vi "N5700 Error Query.vi"(0 "VISA":refnum<visa-resource-name>, 11 "error":errorcluster) -> (4 "VISA out":refnum<visa-resource-name>, 8 "Error Number":i32, 10 "Error Message":string, 15 "error out":errorcluster)   [LabVIEW 2020]
doc: "This VI reads an error code and a message from the instrument's error queue (query SYST:ERR?\"). The instrument error is cast to be within the range allowed for VISA custom errors. See \"Agilent N5700 Readme.html\" file for description of custom error codes\n\nNote: This VI is called automatically by most driver VIs so it is not usually necessary to call this in an application."
panel:
  # "Agilent Technologies  \nSeries N5700A\n  DC Power Supplies"
  # "Read\n  SYSTEM:ERROR?"
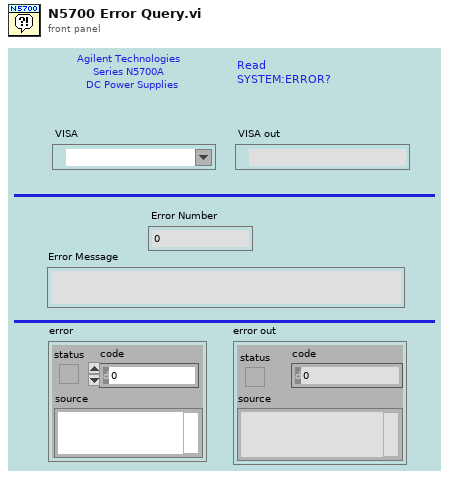
[diagram p1: front panel]
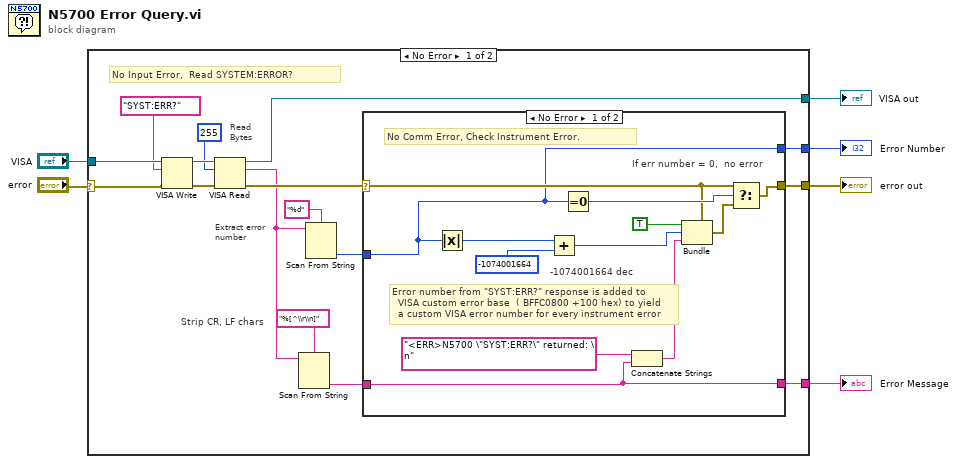
[diagram p0: block diagram]
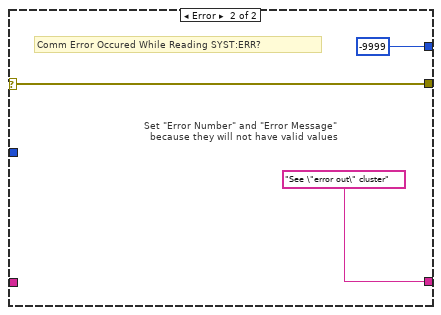
[diagram p2: hidden frame]
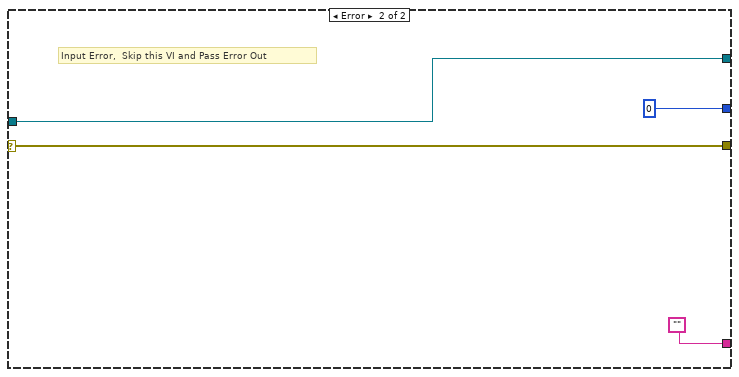
[diagram p3: hidden frame]
diagram:
  n1 = case shown="No Error" "error" {
    selector: "error" -> [w7 w38]
    tunnel: [w22 ""] -> w6
    tunnel: [w21 0] -> w5
    tunnel: [w20 w41] -> w4
    tunnel: "VISA" -> [w19 w41]
    tunnel: [w8 w38] -> w2
    frame No Error {
      # "No Input Error,  Read SYSTEM:ERROR?"
      # "Extract error\nnumber"
      # "Read\nBytes"
      # "Strip CR, LF chars"
      n2 = VISA Write(VISA resource name=w19, write buffer="SYST:ERR?", error in (no error)=w7) -> (VISA resource name out=w18:refnum<visa-resource-name>, error out=w16:errorcluster)  [unwired: 1 out]
      n3 = VISA Read(VISA resource name=w18, byte count=u32 255 ("byte count (0)"), error in (no error)=w16) -> (VISA resource name out=w20:refnum<visa-resource-name>, read buffer=w10:string, error out=w13:errorcluster)  [unwired: 1 out]
      n4 = Scan From String(format string="%[^\\r\\n]", input string=w10) -> (output 1=w9:string)  [unwired: 3 in, 3 out]
      n5 = Scan From String(format string="%d", input string=w10) -> (output 1=w14:i32)  [unwired: 3 in, 3 out]
      n6 = case shown="No Error" w13 {
        selector: w13 -> [w27 w36]
        tunnel: [w31 w36] -> w8
        tunnel: [w28 "See \"error out\" cluster" ("format string")] -> w22
        tunnel: [w26 -9999] -> w21
        tunnel: w14 -> [w26 _]
        tunnel: w9 -> [w28 _]
        frame No Error {
          # "No Comm Error, Check Instrument Error."
          # "Error number from \"SYST:ERR?\" response is added to \n  VISA custom error base  ( BFFC0800 +100 hex) to yield  \n  a custom VISA error number for every instrument error"
          # "-1074001664 dec"
          # "If err number = 0,  no error"
          n7 = Absolute Value(x=w26) -> (abs(x)=w25:i32)
          n8 = Add(x=w25, y=-1074001664) -> (x+y=w23:i32)
          n9 = Equal To 0?(x=w26) -> (x = 0?=w29:bool)
          n10 = Concatenate Strings("<ERR>N5700 \"SYST:ERR?\" returned: \n" ("Source"), w28) -> (w33:string)
          n11 = Bundle(cluster=w27, "status"=TRUE ("Status"), "code"=w23, "source"=w33) -> (w32:errorcluster)
          n12 = Select(t=w27, s=w29, f=w32) -> (s? t:f=w31:errorcluster)
        }
        frame Error {
          # "Set \"Error Number\" and \"Error Message\"\n  because they will not have valid values"
          # "Comm Error Occured While Reading SYST:ERR?"
        }
      }
    }
    frame Error {
      # "Input Error,  Skip this VI and Pass Error Out"
    }
  }
  "Error Message" <- w6
  "Error Number" <- w5
  "VISA out" <- w4
  "error out" <- w2
